vi "RotatorANRv51Monitor.vi"() -> ()   [LabVIEW 2019]
uses:
  Utility/Monitor Communication/Rotator ANRv51/ANRv51_Cluster.ctl
  Instrument_Setup.vi
panel:
  in  "stop":bool
  out "ANRv51":T1
  # "deg"
  # "deg"
  # "V"
  # "Hz"
  # "Rotator ANRv51"
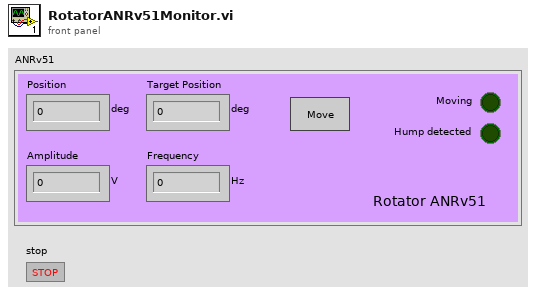
[diagram p1: front panel]
types:
  T1 = typedef "ANRv51_Cluster.ctl" = cluster{"Position":dbl, "Moving":bool, "Hump detected":bool, "Go to Position":bool, "Target Position":dbl, "Amplitude":dbl, "Frequency":dbl}
  T2 = cluster{"error ":bool, "error number":i32, "error code":string}
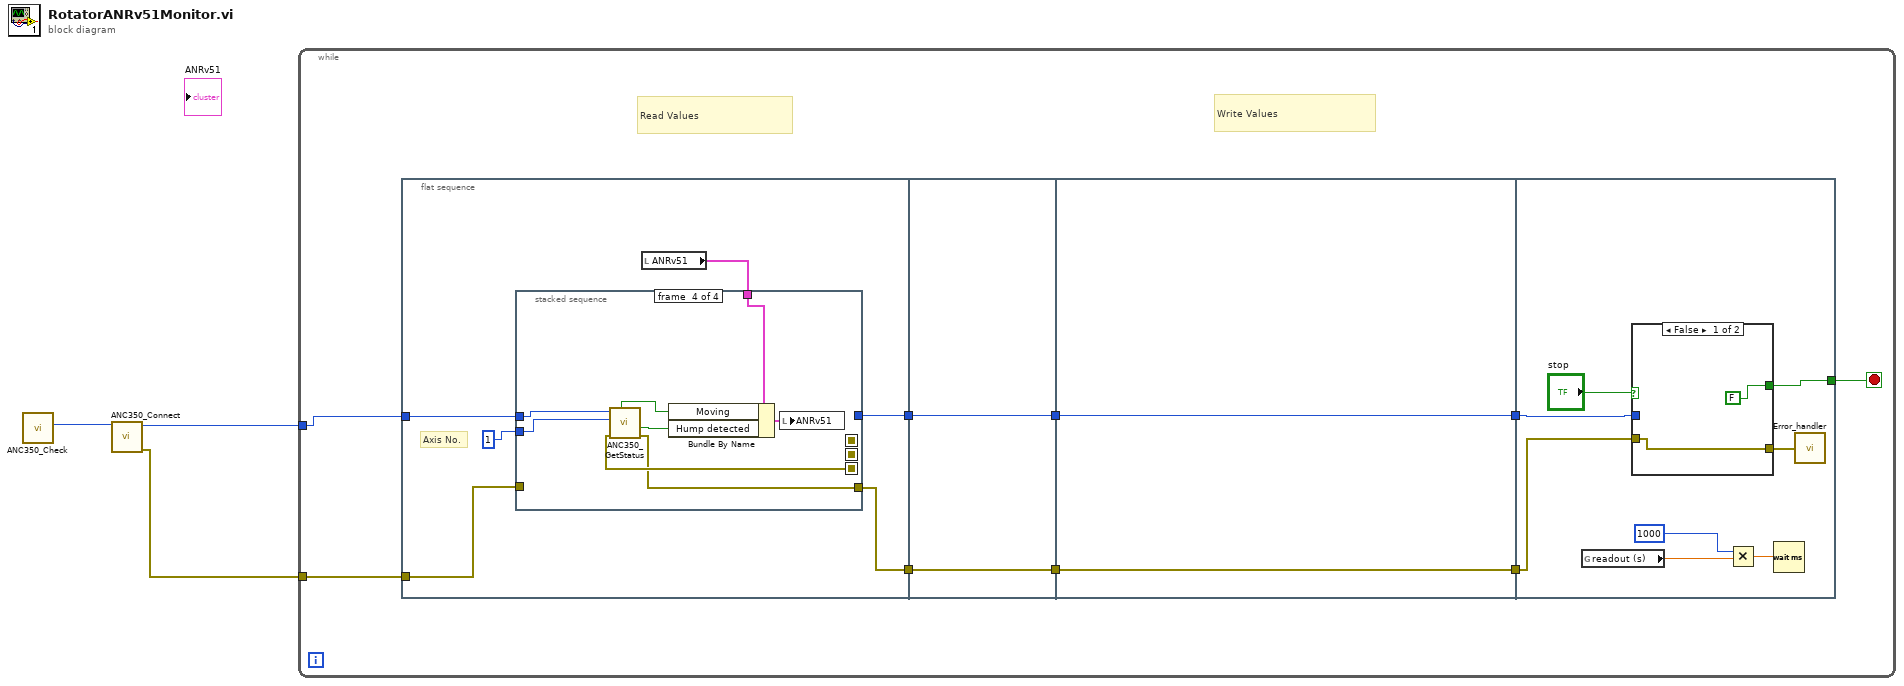
[diagram p0: block diagram]
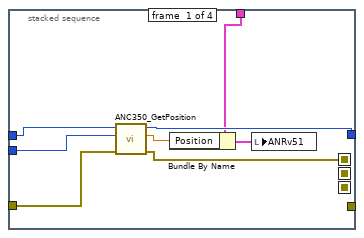
[diagram p2: hidden frame]
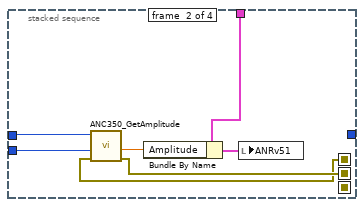
[diagram p3: hidden frame]
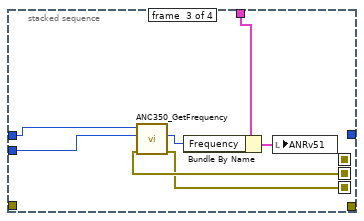
[diagram p4: hidden frame]
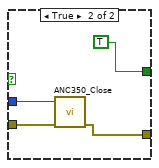
[diagram p5: hidden frame]
diagram:
  n1 = call "ANC350_Check.vi"() -> ("ANC350 found"=w1:i32)  [unwired: 6 in, 1 out]
  n2 = call "ANC350_Connect.vi"("device no"=w1) -> ("error out"=w3:T2, "handle"=w2:i32)  [unwired: 5 in]
  n3 = while {
    tunnel: w3 -> [w11]
    tunnel: w2 -> [w10]
    stop <- w12 stop-if-true
    # "Read Values"
    # "Write Values"
    n4 = flat-sequence {
      tunnel: w11 -> [w17]
      tunnel: w10 -> [w18]
      tunnel: [w15] -> w7
      tunnel: [w14] -> w6
      tunnel: [w50] -> w8
      tunnel: w7 -> [w50]
      tunnel: w6 -> [w49]
      tunnel: [w49] -> w4
      tunnel: [w52] -> w9
      tunnel: w8 -> [w52]
      tunnel: [w51] -> w5
      tunnel: w4 -> [w51]
      tunnel: [w60] -> w12
      tunnel: w9 -> [w55]
      tunnel: w5 -> [w54]
      frame #0 {
        # "Axis No."
        n5 = local read "ANRv51"() -> (w16:T1)
        n6 = stacked-sequence {
          seq-local: [_ w28 _ _] -> [_ _ w38 _]
          seq-local: [w22 _ _ _] -> [_ w27 _ _]
          seq-local: [_ _ w34 _] -> [_ _ _ w43]
          tunnel: w18 -> [w26 w33 w40 w48]
          tunnel: w17 -> [w24 _ _ _]
          tunnel: w16 -> [w20 w31 w36 w46]
          tunnel: [w23 _ _ _] -> w15
          tunnel: [_ _ _ w42] -> w14
          tunnel: 1 -> [w25 w29 w39 w47]
          frame #0 {
            n7 = call "ANC350_GetPosition.vi"("error in"=w24, "axis no"=w25, "device handle"=w26) -> ("error out"=w22:T2, "position [µm/°/m°]"=w21:dbl, "device handle Out"=w23:i32)  [unwired: 2 in]
            n8 = Bundle By Name(cluster=w20, "Position"=w21) -> (w19:T1)
            n9 = local write "ANRv51"(w19) -> ()
          }
          frame #1 {
            n10 = call "ANC350_GetAmplitude.vi"("error in"=w27, "axis no"=w29, "device handle"=w33) -> ("error out"=w28:T2, "amplitude [V]"=w32:dbl)  [unwired: 2 in, 1 out]
            n11 = Bundle By Name(cluster=w31, "Amplitude"=w32) -> (w30:T1)
            n12 = local write "ANRv51"(w30) -> ()
          }
          frame #2 {
            n13 = call "ANC350_GetFrequency.vi"("error in"=w38, "axis no"=w39, "device handle"=w40) -> ("error out"=w34:T2, "PositionerFrequency [Hz]"=w37:i32)  [unwired: 2 in, 1 out]
            n14 = Bundle By Name(cluster=w36, "Frequency"=w37) -> (w35:T1)
            n15 = local write "ANRv51"(w35) -> ()
          }
          frame #3 {
            n16 = call "ANC350_GetStatus.vi"("error in"=w43, "axis no"=w47, "device handle"=w48) -> ("error out"=w42:T2, "stop detected"=w45:bool, "moving"=w44:bool)  [unwired: 1 in, 2 out]
            n17 = Bundle By Name(cluster=w46, "Moving"=w44, "Hump detected"=w45) -> (w41:T1)
            n18 = local write "ANRv51"(w41) -> ()
          }
        }
      }
      frame #1 {
      }
      frame #2 {
      }
      frame #3 {
        n19 = global read "Instrument_Setup.vi" "readout (s)"() -> (w58:dbl)
        n20 = case shown="False" "stop" {
          tunnel: [FALSE TRUE] -> w60
          tunnel: w55 -> [_ w65]
          tunnel: w54 -> [w61 w64]
          tunnel: [w61 w63] -> w53
          frame False {
          }
          frame True {
            n21 = call "ANC350_Close.vi"("error in"=w64, "device handle"=w65) -> ("error out"=w63:T2)  [unwired: 5 in]
          }
        }
        n22 = Multiply(x=1000, y=w58) -> (x*y=w57:dbl)
        n23 = Wait (ms)(milliseconds to wait=w57) -> ()  [unwired: 1 out]
        n24 = call "Error_handler.vi"("error constant"=w53) -> ()
      }
    }
  }
